vi "ATF Storage-AO Data FGV.vi"(7 "Option":T1(ring)=enum."Read 1", 8 "error in (no error)":errorcluster, 9 "Time Stamp In":timestamp, 10 "AO Channel Names":string[](array[string]), 11 "AO Values In":dbl[](array[numeric])) -> (0 "error out":errorcluster, 1 "AO Channel Names":string[](array[string]), 2 "All data out":waveform(dbl)[](array[waveform]), 3 "AO Values Out":dbl[](array[numeric]), 4 "Time Stamp Out":timestamp)   [LabVIEW 2022 SP3]
uses:
  RT Controls/ATF Storage-FGV Read write.ctl
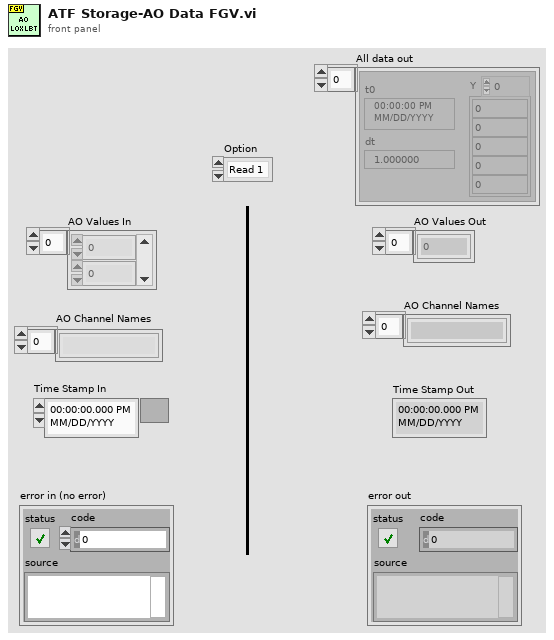
[diagram p1: front panel]
types:
  T1 = enum16{"Init", "Read", "Write 'All'", "Write 'n'", "Write Safe Value", "Write Start Time", "Read 1"}
  T2 = typedef "ATF Storage-FGV Read write.ctl" = enum16{"Write", "Read"}
  T3 = cluster{"Samples to Read":i32, "Pattern Mode?":bool, "dt(sec)":dbl, "DO Init Time (Samples)":i32, "dt per Read/Write":dbl, "Write Pointer":i32, "Pattern Size":i32, "Loop Rate (mSec)":i32, "Buffer Size (Samples)":i32, "Sampling rate":dbl, "Max DO Delay Time (samples)":dbl, "Min DO Delay Time (samples)":dbl, "Queue Size":i32, "DO Init Sample Duration (Sec)":dbl}
  T4 = cluster{"AO Channel Names":string[], "AO Safe Waveform":waveform(dbl)[], "dt per Read/Write":dbl, "AO Safe Value":dbl[]}
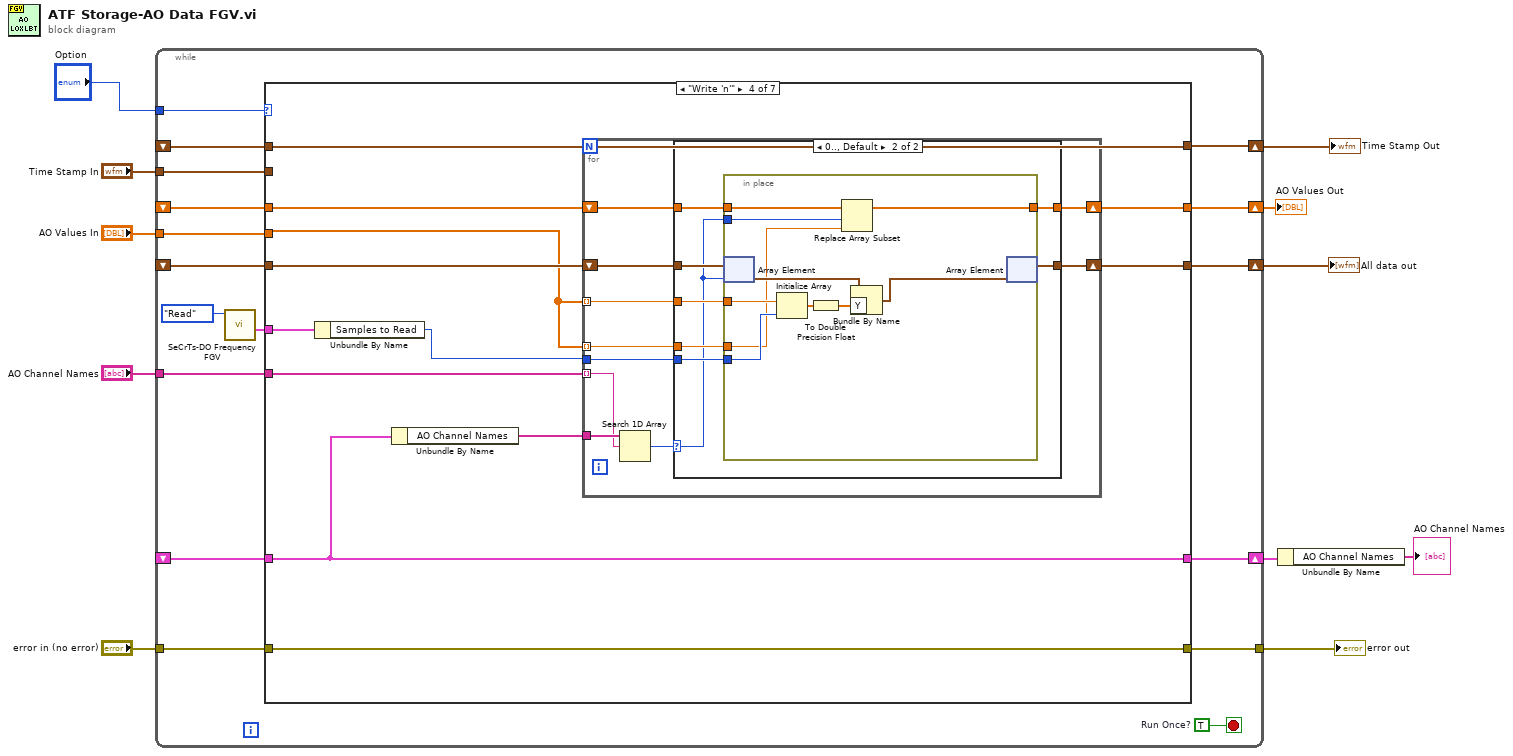
[diagram p0: block diagram]
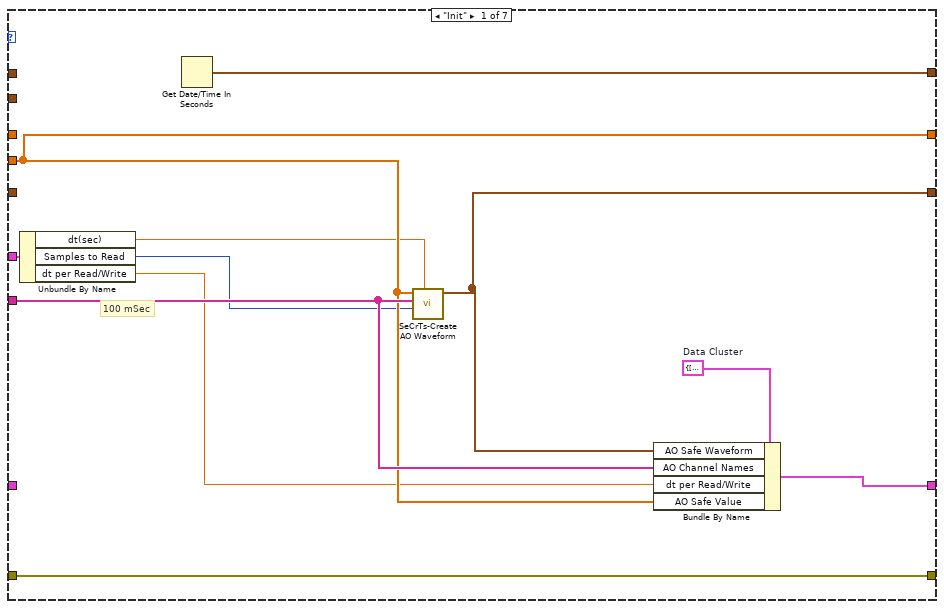
[diagram p2: hidden frame]
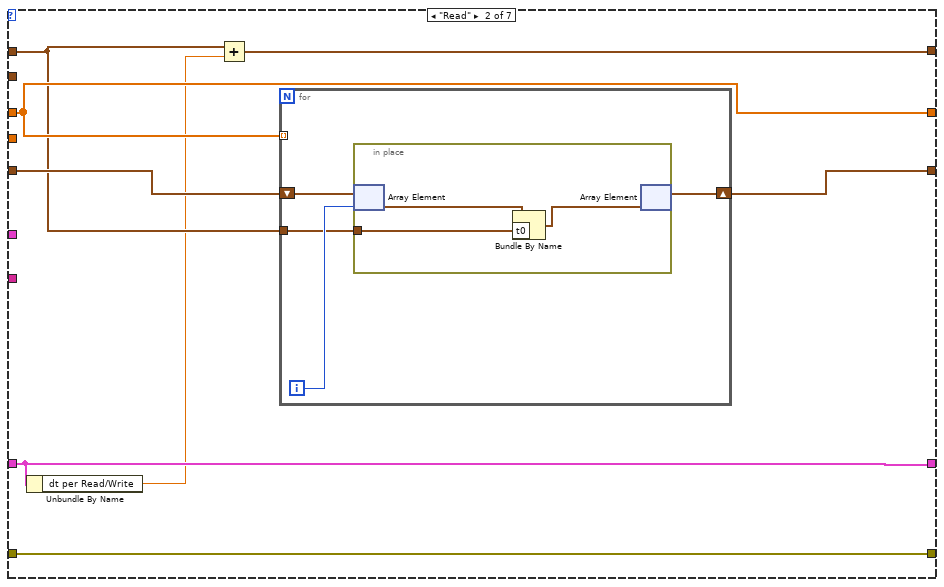
[diagram p3: hidden frame]
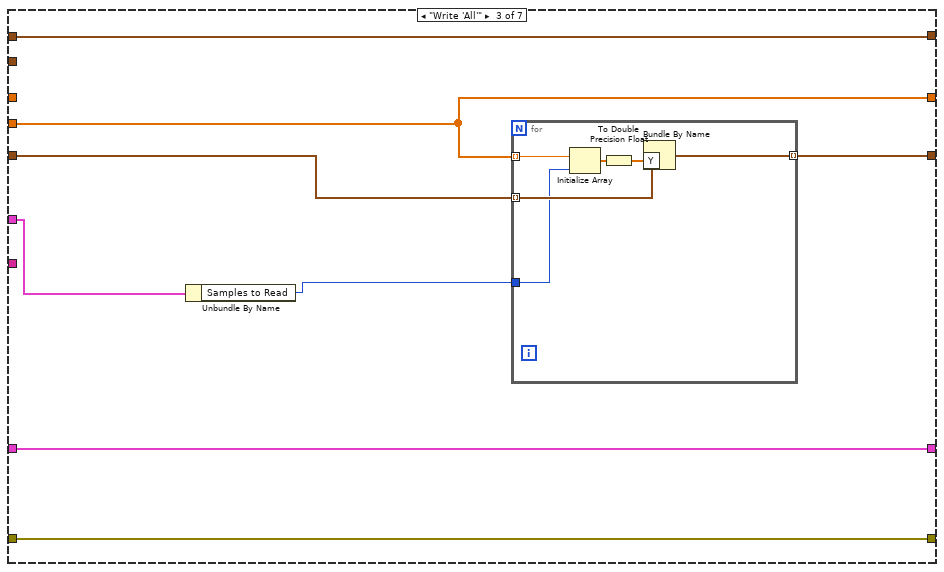
[diagram p4: hidden frame]
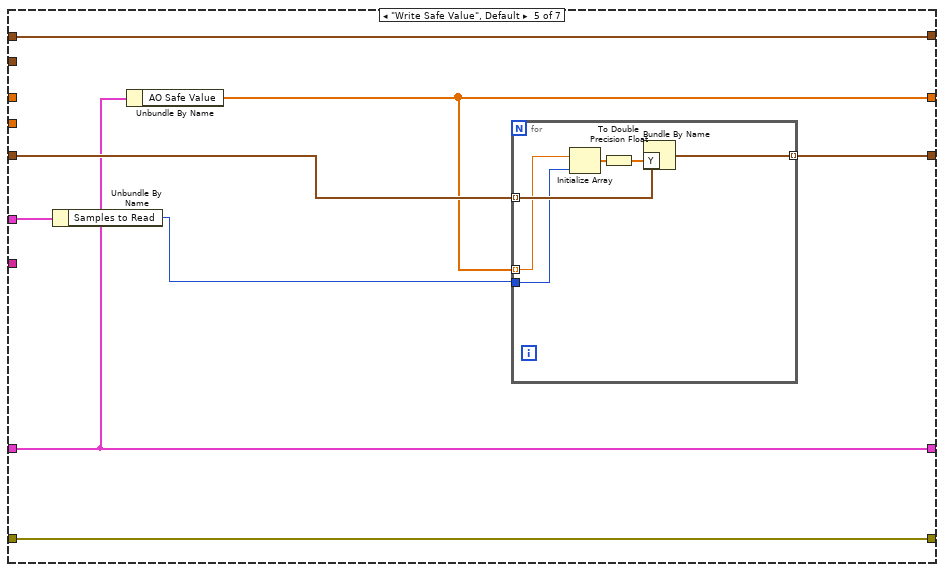
[diagram p6: hidden frame]
diagram:
  n1 = while {
    tunnel: "AO Values In" -> [w26]
    shift-right: [w27] -> w3
    shift-left: _ -> [w25]
    shift-right: [w24] -> w10
    shift-left: _ -> [w23]
    shift-right: [w22] -> w9
    shift-left: _ -> [w21]
    shift-right: [w20] -> w2
    shift-left: _ -> [w19]
    tunnel: "error in (no error)" -> [w18]
    tunnel: [w17] -> w7
    tunnel: "AO Channel Names" -> [w16]
    tunnel: "Time Stamp In" -> [w15]
    tunnel: "Option" -> [w14]
    stop <- w28 stop-if-true
    w28 = TRUE  # Run Once?
    n2 = call "SeCrTs-DO Frequency  FGV.vi"("Write/Read"=ATF_Storage-FGV_Read_write."Read") -> ("DO Set Frequency (R)"=w12:T3)  [unwired: 9 in, 1 out]
    n3 = case shown="\"Write 'n'\"" w14 {
      tunnel: [w33 w43 w57 w72 w113 w129 w134] -> w27
      tunnel: w26 -> [w33 _ w57 w71 _ _ _]
      tunnel: w25 -> [_ w43 _ w73 _ w129 w134]
      tunnel: [w39 w41 w62 w80 w118 w125 w130] -> w24
      tunnel: w23 -> [_ w42 w62 w80 w118 _ w130]
      tunnel: [w34 w44 w58 w77 w115 w128 w131] -> w22
      tunnel: w21 -> [_ w46 w59 w78 w116 w128 w131]
      tunnel: [w36 w45 w61 w75 w114 w127 w133] -> w20
      tunnel: w19 -> [_ w45 w61 w75 w114 w127 w133]
      tunnel: w18 -> [w37 w47 w60 w79 w117 w126 w132]
      tunnel: [w37 w47 w60 w79 w117 w126 w132] -> w17
      tunnel: w16 -> [w35 _ _ w76 _ _ _]
      tunnel: w15 -> [_ _ _ _ _ w125 _]
      tunnel: w12 -> [w32 _ w56 w70 w112 _ _]
      frame "Init" {
        w38 = T4 {"AO Channel Names"=[], "AO Safe Waveform"=[], "dt per Read/Write"=100.0, "AO Safe Value"=[]}  # Data Cluster
        # "100 mSec"
        n4 = Unbundle By Name(w32) -> ("dt(sec)"=w29:dbl, "Samples to Read"=w31:i32, "dt per Read/Write"=w30:dbl)
        n5 = Get Date/Time In Seconds() -> (seconds since 1Jan1904=w39:timestamp)
        n6 = call "SeCrTs-Create AO Waveform.vi"("dt(sec)"=w29, "Size"=w31, "AO Channel Names"=w35, "AO Values In"=w33) -> ("AO Waveform"=w34:waveform(dbl)[])  [unwired: 7 in]
        n7 = Bundle By Name(cluster=w38, "AO Safe Waveform"=w34, "AO Channel Names"=w35, "dt per Read/Write"=w30, "AO Safe Value"=w33) -> (w36:T4)
      }
      frame "Read" {
        n8 = Unbundle By Name(w45) -> ("dt per Read/Write"=w40:dbl)
        n9 = Add(x=w42, y=w40) -> (x+y=w41:timestamp)
        n10 = for {
          shift-right: [w50] -> w44
          shift-left: w46 -> [w51]
          tunnel: w42 -> [w48]
          tunnel: w43 -> [_] mode=indexing
          i -> [w49]
          n11 = in-place {
            in-place-border: w48 -> [w52]
            n12 = in-place-array #1(w51, w49) -> (w54:waveform(dbl))
            n13 = Bundle By Name(cluster=w54, "t0"=w52) -> (w53:waveform(dbl))
            n14 = in-place-array #1(w53) -> (w50:waveform(dbl)[])  [unwired: 1 out]
          }
        }
      }
      frame "Write 'All'" {
        n15 = Unbundle By Name(w56) -> ("Samples to Read"=w55:i32)
        n16 = for {
          tunnel: w57 -> [w67] mode=indexing
          tunnel: [w68] -> w58 mode=indexing
          tunnel: w55 -> [w63]
          tunnel: w59 -> [w64] mode=indexing
          n17 = Initialize Array(w67, w63) -> (w66:dbl[])
          n18 = To Double Precision Float(number=w66) -> (double precision float=w65:dbl[])
          n19 = Bundle By Name(cluster=w64, "Y"=w65) -> (w68:waveform(dbl))
        }
      }
      frame "Write 'n'" {
        n20 = Unbundle By Name(w70) -> ("Samples to Read"=w69:i32)
        n21 = Unbundle By Name(w75) -> ("AO Channel Names"=w74:string[])
        n22 = for {
          tunnel: w71 -> [w89] mode=indexing
          tunnel: w69 -> [w87]
          tunnel: w71 -> [w88] mode=indexing
          tunnel: w76 -> [w85] mode=indexing
          tunnel: w74 -> [w86]
          shift-right: [w90] -> w77
          shift-left: w78 -> [w83]
          shift-right: [w81] -> w72
          shift-left: w73 -> [w82]
          n23 = Search 1D Array(1D array=w86, element=w85) -> (index of element=w84:i32)  [unwired: 1 in]
          n24 = case shown="0.., Default" w84 {
            selector: w84 -> [_ w93]
            tunnel: [w92 w96] -> w90
            tunnel: w89 -> [_ w100]
            tunnel: w88 -> [_ w99]
            tunnel: w87 -> [_ w98]
            tunnel: w83 -> [w92 w97]
            tunnel: w82 -> [w91 w95]
            tunnel: [w91 w94] -> w81
            frame -1 {
            }
            frame 0.., Default {
              n25 = in-place {
                in-place-border: w100 -> [w110]
                in-place-border: w99 -> [w101]
                in-place-border: w98 -> [w107]
                in-place-border: w95 -> [w104]
                in-place-border: [w103] -> w94
                in-place-border: w93 -> [w102]
                n26 = in-place-array #2(w97, w93) -> (w105:waveform(dbl))
                n27 = Initialize Array(w110, w107) -> (w109:dbl[])
                n28 = To Double Precision Float(number=w109) -> (double precision float=w108:dbl[])
                n29 = Replace Array Subset(array=w104, new element=w101, index=w102) -> (w103:dbl[])
                n30 = Bundle By Name(cluster=w105, "Y"=w108) -> (w106:waveform(dbl))
                n31 = in-place-array #2(w106) -> (w96:waveform(dbl)[])  [unwired: 1 out]
              }
            }
          }
        }
      }
      frame "Write Safe Value", Default {
        n32 = Unbundle By Name(w112) -> ("Samples to Read"=w111:i32)
        n33 = Unbundle By Name(w114) -> ("AO Safe Value"=w113:dbl[])
        n34 = for {
          tunnel: [w124] -> w115 mode=indexing
          tunnel: w111 -> [w120]
          tunnel: w116 -> [w121] mode=indexing
          tunnel: w113 -> [w119] mode=indexing
          n35 = Initialize Array(w119, w120) -> (w123:dbl[])
          n36 = To Double Precision Float(number=w123) -> (double precision float=w122:dbl[])
          n37 = Bundle By Name(cluster=w121, "Y"=w122) -> (w124:waveform(dbl))
        }
      }
      frame "Write Start Time" {
      }
      frame "Read 1" {
      }
    }
  }
  "error out" <- w7
  "Time Stamp Out" <- w10
  "All data out" <- w9
  "AO Values Out" <- w3
  n38 = Unbundle By Name(w2) -> ("AO Channel Names"=→"AO Channel Names":string[])
